vi "nanoVoltRead_withTemp.vi"() -> ()   [LabVIEW 2013]
uses:
  <vilib>/Utility/file.llb/Write To Spreadsheet File (string).vi
panel:
  in  "Previous Top T":dbl
  in  "Temp Rate (s)":dbl=0.25
  in  "Previous Delta T":dbl
  in  "T read time":dbl
  out "Temp2 (C)":dbl format="%#.4g"
  out "Temp1 (C)":dbl format="%#.4g"
  out "Delta T (C)":dbl format="%#.4g"
  in  "Temp2 Port":tag="Dev2"
  in  "Temp1 Port":tag="Dev1"
  in  "Rate (0.1 - 5)":string="5"
  out "Time (s)":dbl caption="Elapsed Time (s)"
  out "XY Graph":cluster{dbl[], dbl[]}[](graph)
  in  "file (use dialog)":path=path "C:/VNA-FMR user/Desktop/nanoVolt"
  out "Measurement Number":i32
  in  "stop":bool
  out "Voltage(V)":dbl
  in  "GPIB\nAddress":string="9"
  # "Keithley Model 2182A Nanovoltmeter Read\n12/13/2013\nMichael Kabatek & David Ellsworth\nCSU Magnetics Lab"
  # "Ignore These"
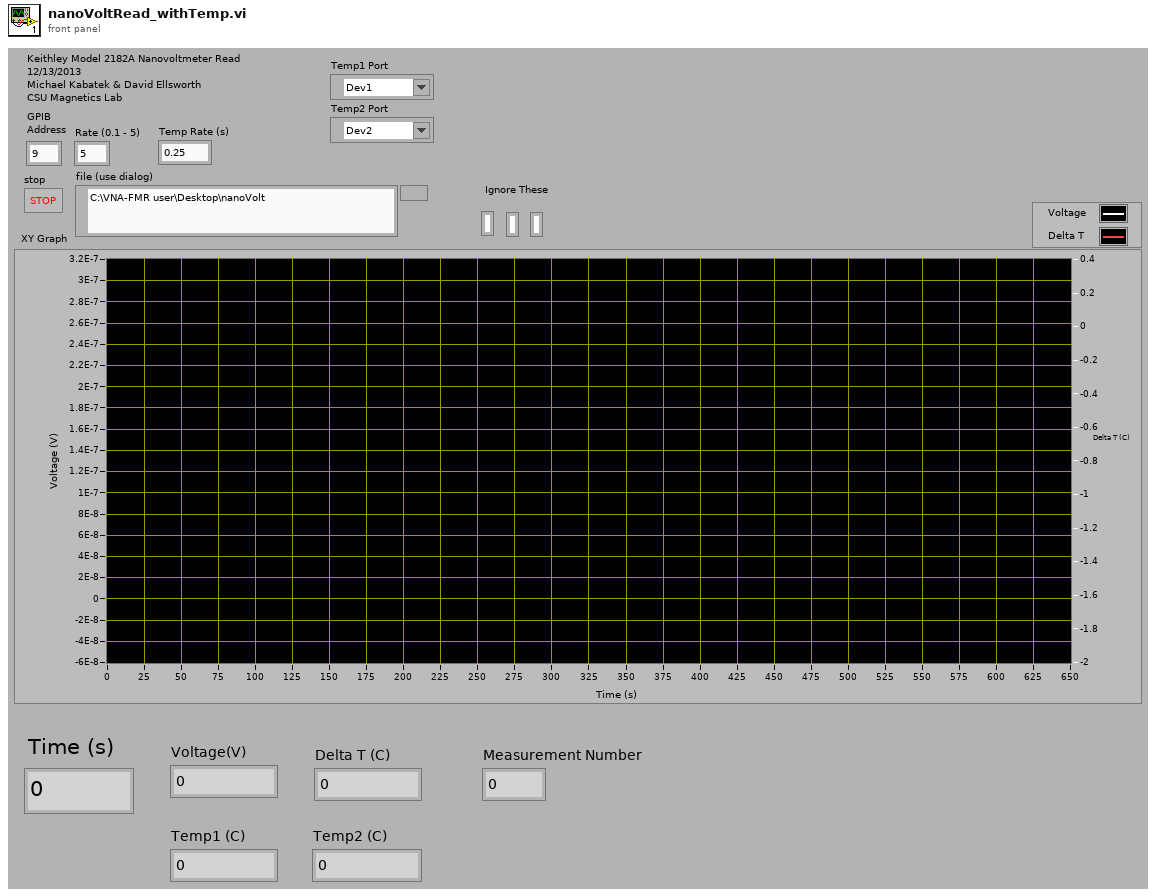
[diagram p1: front panel]
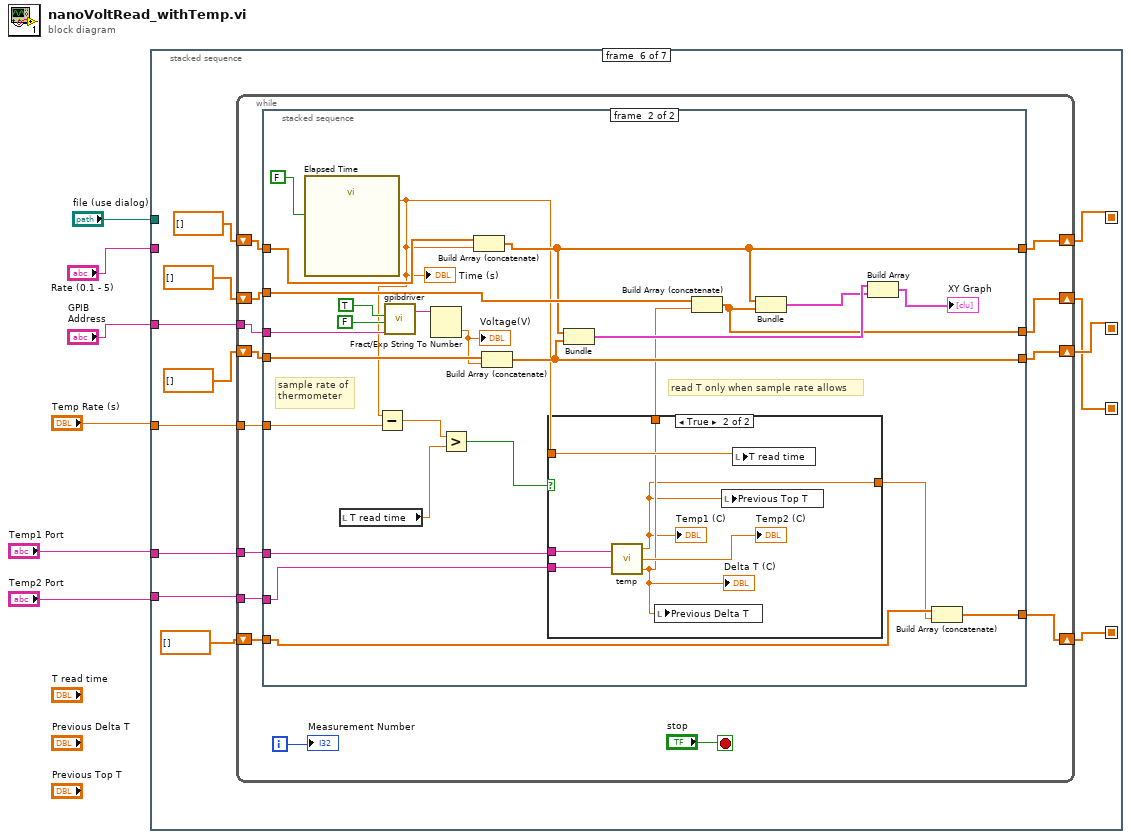
[diagram p0: block diagram]
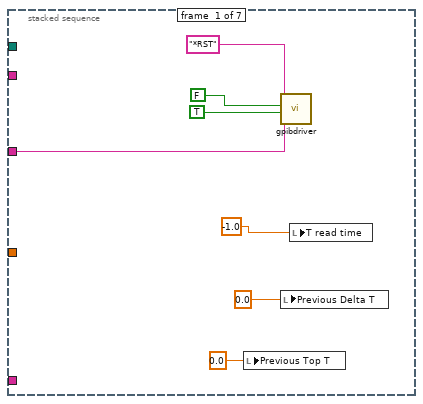
[diagram p2: hidden frame]
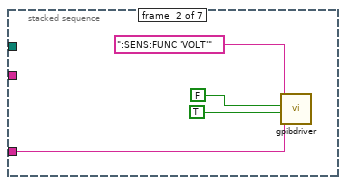
[diagram p3: hidden frame]
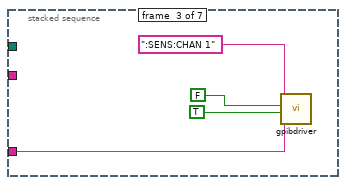
[diagram p4: hidden frame]
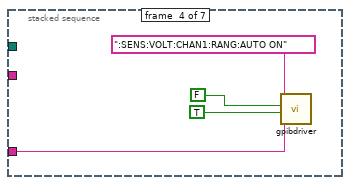
[diagram p5: hidden frame]
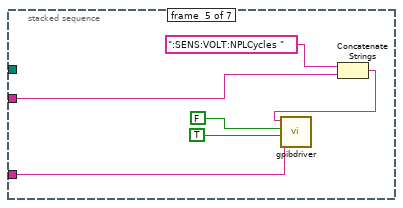
[diagram p6: hidden frame]
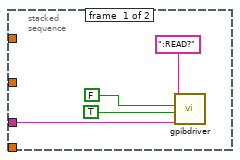
[diagram p7: hidden frame]
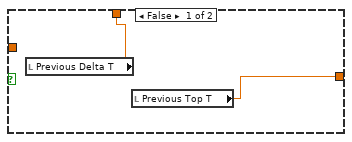
[diagram p8: hidden frame]
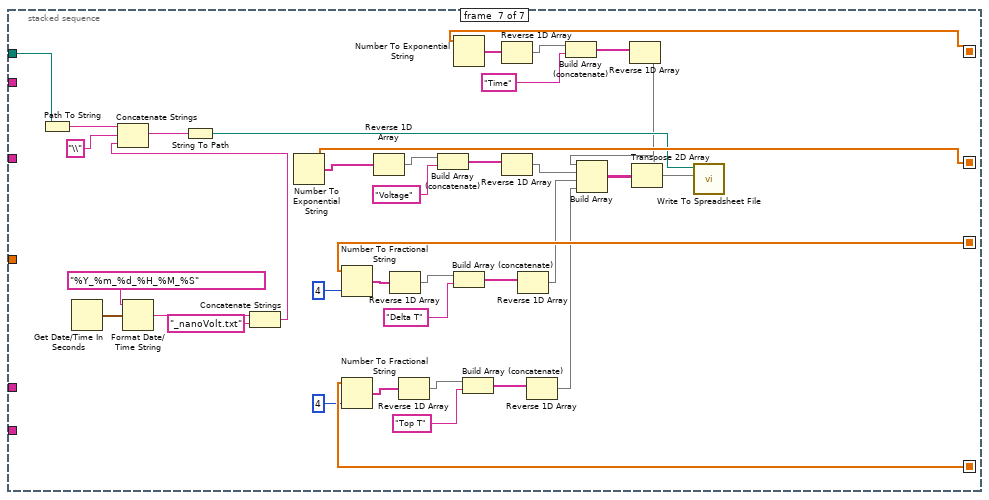
[diagram p9: hidden frame]
diagram:
  n1 = stacked-sequence {
    seq-local: [_ _ _ _ _ w41 _] -> [_ _ _ _ _ _ w124]
    seq-local: [_ _ _ _ _ w39 _] -> [_ _ _ _ _ _ w117]
    seq-local: [_ _ _ _ _ w36 _] -> [_ _ _ _ _ _ w121]
    seq-local: [_ _ _ _ _ w33 _] -> [_ _ _ _ _ _ w119]
    tunnel: "GPIB\nAddress" -> [w10 w14 w18 w22 w29 w43 _]
    tunnel: "file (use dialog)" -> [_ _ _ _ _ _ w126]
    tunnel: "Temp1 Port" -> [_ _ _ _ _ w38 _]
    tunnel: "Temp2 Port" -> [_ _ _ _ _ w37 _]
    tunnel: "Rate (0.1 - 5)" -> [_ _ _ _ w26 _ _]
    tunnel: "Temp Rate (s)" -> [_ _ _ _ _ w34 _]
    frame #0 {
      n2 = local write "Previous Top T"(0.0 ("Previous Top T")) -> ()
      n3 = call "gpibdriver.vi"("Characters to Write"="*RST", "Read"=FALSE, "Write"=TRUE ("Write 3"), "GPIB\nAddress"=w10) -> ()  [unwired: 2 in, 1 out]
      n4 = local write "Previous Delta T"(0.0 ("Previous T")) -> ()
      n5 = local write "T read time"(-1.0 ("read T")) -> ()
    }
    frame #1 {
      n6 = call "gpibdriver.vi"("Characters to Write"=":SENS:FUNC 'VOLT'", "Read"=FALSE, "Write"=TRUE ("Write 3"), "GPIB\nAddress"=w14) -> ()  [unwired: 2 in, 1 out]
    }
    frame #2 {
      n7 = call "gpibdriver.vi"("Characters to Write"=":SENS:CHAN 1", "Read"=FALSE, "Write"=TRUE ("Write 3"), "GPIB\nAddress"=w18) -> ()  [unwired: 2 in, 1 out]
    }
    frame #3 {
      n8 = call "gpibdriver.vi"("Characters to Write"=":SENS:VOLT:CHAN1:RANG:AUTO ON", "Read"=FALSE, "Write"=TRUE ("Write 3"), "GPIB\nAddress"=w22) -> ()  [unwired: 2 in, 1 out]
    }
    frame #4 {
      n9 = Concatenate Strings(":SENS:VOLT:NPLCycles " ("Characters to Write"), w26) -> (w27:string)
      n10 = call "gpibdriver.vi"("Characters to Write"=w27, "Read"=FALSE, "Write"=TRUE ("Write 3"), "GPIB\nAddress"=w29) -> ()  [unwired: 2 in, 1 out]
    }
    frame #5 {
      n11 = while {
        tunnel: w43 -> [w57]
        shift-right: [w55] -> w41
        shift-left: dbl[] [] -> [w54]
        shift-right: [w51] -> w39
        shift-left: dbl[] [] -> [w52]
        tunnel: w38 -> [w50]
        tunnel: w37 -> [w49]
        shift-right: [w48] -> w36
        shift-left: dbl[] [] -> [w47]
        tunnel: w34 -> [w46]
        shift-right: [w44] -> w33
        shift-left: dbl[] [] -> [w45]
        i -> [w53]
        stop <- "stop" stop-if-true
        n12 = stacked-sequence {
          tunnel: w57 -> [w58 w85]
          tunnel: [_ w79] -> w55
          tunnel: w54 -> [_ w84]
          tunnel: w52 -> [_ w81]
          tunnel: [_ w71] -> w51
          tunnel: w50 -> [_ w78]
          tunnel: w49 -> [_ w77]
          tunnel: [_ w73] -> w48
          tunnel: w47 -> [_ w74]
          tunnel: w46 -> [_ w65]
          tunnel: w45 -> [_ w64]
          tunnel: [_ w62] -> w44
          frame #0 {
            n13 = call "gpibdriver.vi"("Characters to Write"=":READ?", "Read"=FALSE, "Write"=TRUE ("Write 3"), "GPIB\nAddress"=w58) -> ()  [unwired: 2 in, 1 out]
          }
          frame #1 {
            # "read T only when sample rate allows"
            # "sample rate of\nthermometer"
            n14 = call "Elapsed Time"("Auto Reset"=FALSE) -> ("Elapsed Time (s)"=w68:dbl)  [unwired: 11 in, 7 out]
            "Time (s)" <- w68
            n15 = local read "T read time"() -> (w66:dbl)
            n16 = Subtract(x=w68, y=w65) -> (x-y=w67:dbl)
            n17 = call "gpibdriver.vi"("Read"=TRUE, "Write"=FALSE ("Write 3"), "GPIB\nAddress"=w85) -> ("Characters Read"=w82:string)  [unwired: 3 in]
            n18 = Fract/Exp String To Number(string=w82) -> (number=w83:dbl)  [unwired: 3 in, 1 out]
            "Voltage(V)" <- w83
            n19 = Greater?(x=w67, y=w66) -> (0:w69:bool)
            n20 = Build Array (concatenate)(w81, w68) -> (w71:dbl[])
            n21 = Build Array (concatenate)(w84, w83) -> (w79:dbl[])
            n22 = case shown="True" w69 {
              tunnel: w78 -> [_ w95]
              tunnel: w77 -> [_ w94]
              tunnel: [w89 w91] -> w75
              tunnel: w68 -> [_ w92]
              tunnel: [w88 w90] -> w63
              frame False {
                n23 = local read "Previous Delta T"() -> (w89:dbl)
                n24 = local read "Previous Top T"() -> (w88:dbl)
              }
              frame True {
                n25 = call "temp.vi"("Temp1 (Top) Port"=w95, "Temp2 (Bottom) Port"=w94) -> ("Top"=w90:dbl, "Bottom"=→"Temp2 (C)":dbl, "Delta T"=w91:dbl)
                "Delta T (C)" <- w91
                "Temp1 (C)" <- w90
                n26 = local write "Previous Delta T"(w91) -> ()
                n27 = local write "Previous Top T"(w90) -> ()
                n28 = local write "T read time"(w92) -> ()
              }
            }
            n29 = Bundle(w71, w79) -> (w76:cluster{dbl[], dbl[]})  [unwired: 1 in]
            n30 = Build Array (concatenate)(w74, w75) -> (w73:dbl[])
            n31 = Bundle(w71, w73) -> (w70:cluster{dbl[], dbl[]})  [unwired: 1 in]
            n32 = Build Array(w76, w70) -> (→"XY Graph":cluster{dbl[], dbl[]}[])
            n33 = Build Array (concatenate)(w64, w63) -> (w62:dbl[])
          }
        }
        "Measurement Number" <- w53
      }
    }
    frame #6 {
      n34 = Path To String(path=w126) -> (string=w129:string)
      n35 = Get Date/Time In Seconds() -> (seconds since 1Jan1904=w133:timestamp)
      n36 = Format Date/Time String(time format string (%c)="%Y_%m_%d_%H_%M_%S", seconds (now)=w133) -> (date/time string=w131:string)  [unwired: 1 in]
      n37 = Concatenate Strings(w131, "_nanoVolt.txt" ("string")) -> (w125:string)
      n38 = Concatenate Strings(w129, "\\" ("string"), w125) -> (w127:string)
      n39 = String To Path(string=w127) -> (path=w123:path)
      n40 = Number To Exponential String(number=w124) -> (E-format string=w111:string[])  [unwired: 3 in]
      n41 = Number To Fractional String(number=w121, precision (6)=i16 4) -> (F-format string=w106:string[])  [unwired: 2 in]
      n42 = Number To Fractional String(number=w119, precision (6)=i16 4) -> (F-format string=w99:string[])  [unwired: 2 in]
      n43 = Reverse 1D Array(array=w111) -> (reversed array=w110:string[])
      n44 = Reverse 1D Array(array=w106) -> (reversed array=w105:string[])
      n45 = Reverse 1D Array(array=w99) -> (reversed array=w101:string[])
      n46 = Build Array (concatenate)(w110, "Voltage") -> (w109:string[])
      n47 = Number To Exponential String(number=w117) -> (E-format string=w115:string[])  [unwired: 3 in]
      n48 = Build Array (concatenate)(w105, "Delta T") -> (w107:string[])
      n49 = Build Array (concatenate)(w101, "Top T") -> (w102:string[])
      n50 = Reverse 1D Array(array=w115) -> (reversed array=w114:string[])
      n51 = Reverse 1D Array(array=w109) -> (reversed array=w108:string[])
      n52 = Reverse 1D Array(array=w107) -> (reversed array=w104:string[])
      n53 = Reverse 1D Array(array=w102) -> (reversed array=w98:string[])
      n54 = Build Array (concatenate)(w114, "Time") -> (w113:string[])
      n55 = Reverse 1D Array(array=w113) -> (reversed array=w112:string[])
      n56 = Build Array(w112, w108, w104, w98) -> (w116:string[][])
      n57 = Transpose 2D Array(2D array=w116) -> (transposed array=w122:string[][])
      n58 = call-poly <vilib>:"Write To Spreadsheet File.vi"("2D data"=w122, "file path (dialog if empty)"=w123) -> ()  [unwired: 6 in, 1 out]
    }
  }
